vi "Close Connection.vi"(8 "error in":errorcluster, 11 "NetStream in":refnum<class "NetStream.lvclass">) -> (0 "error out":errorcluster, 3 "NetStream out":refnum<class "NetStream.lvclass">)   [LabVIEW 2022 SP3, in "hse-network.lvlib" / "NetStream.lvclass"]
doc: "____\nHAMPEL SOFTWARE ENGINEERING v3.8.0 (2023-12-18 14:41)"
uses:
  NetStream.lvclass
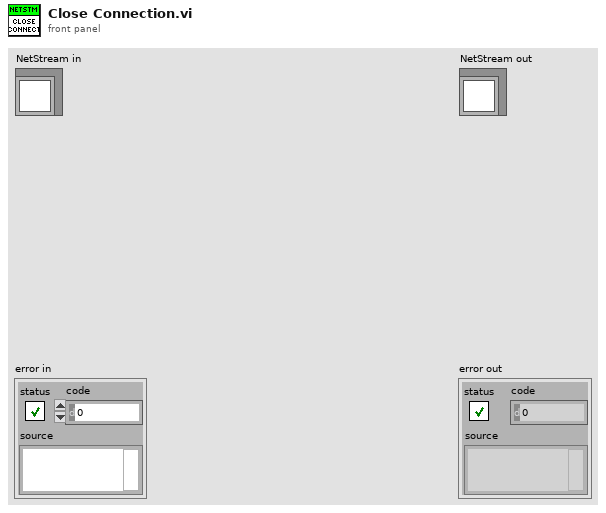
[diagram p1: front panel]
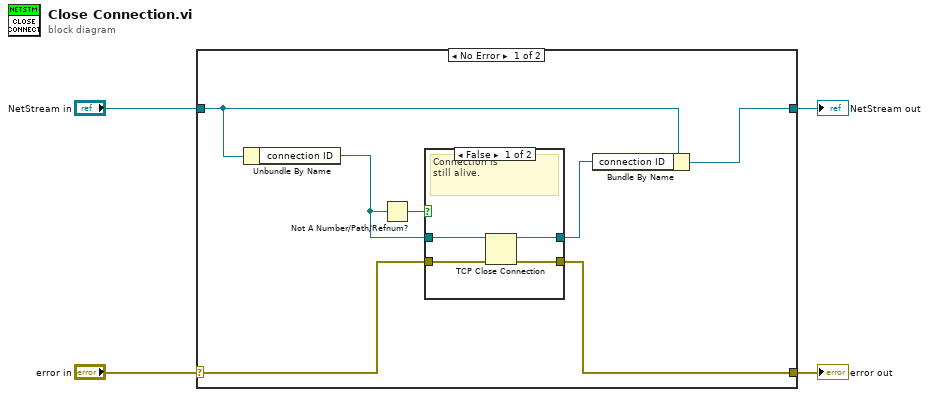
[diagram p0: block diagram]
diagram:
  n1 = case shown="No Error" "error in" {
    selector: "error in" -> [w11 w19]
    tunnel: [w10 w19] -> w3
    tunnel: [w8 w18] -> w1
    tunnel: "NetStream in" -> [w9 w18]
    frame No Error {
      n2 = Unbundle By Name(w9) -> ("connection ID"=w6:refnum<k5>)
      n3 = Not A Number/Path/Refnum?(number/path/refnum=w6) -> (NaN/Path/Refnum?=w5:bool)
      n4 = case shown="False" w5 {
        tunnel: w6 -> [w15 w16]
        tunnel: w11 -> [w14 w17]
        tunnel: [w13 w17] -> w10
        tunnel: [w12 w16] -> w7
        frame False {
          # "Connection is\nstill alive."
          n5 = TCP Close Connection(connection ID=w15, error in (no error)=w14) -> (connection ID out=w12:refnum<k5>, error out=w13:errorcluster)  [unwired: 1 in]
        }
        frame True {
          # "Connection was\nclosed before."
        }
      }
      n6 = Bundle By Name(cluster=w9, "connection ID"=w7) -> (w8:refnum<class "NetStream.lvclass">)
    }
    frame Error {
    }
  }
  "error out" <- w3
  "NetStream out" <- w1
